vi "STD溶解氧_获取温度和测量值.vi"(5 "大气压补偿":dbl=1.0, 7 "盐度补偿":dbl, 8 "error in (no error)":errorcluster caption="错误输入（无错误）", 11 "MB session in":refnum<class "MB_Master.lvclass">) -> (0 "error out":errorcluster caption="错误输出", 2 "输出值":cluster{"温度测量值":sgl, "DO%":sgl, "DOmg/L":sgl}, 3 "MB session out":refnum<class "MB_Master.lvclass">)   [LabVIEW 2016, in "斯坦道多参数.lvlib"]
uses:
  <vilib>/Plasmionique/MB Master/MB_Master/MB_Master.lvclass
  <vilib>/Plasmionique/MB Master/MB Master.lvlib
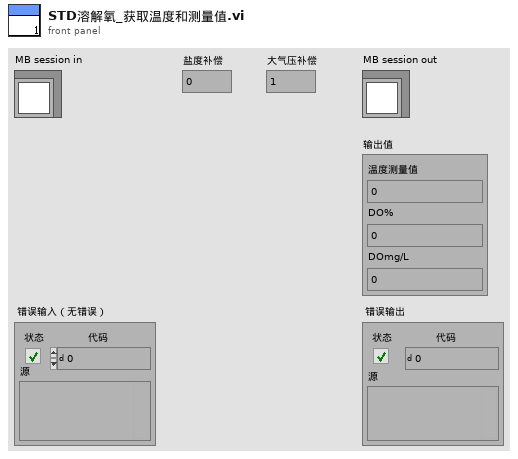
[diagram p1: front panel]
types:
  T1 = cluster{"pH":u32, "DO":u32, "Cond":u32, "Turb":u32, "叶绿素a":u32, "藻密度":u32, "ORP":u32, "COD":u32, "氯化物":u32, "氨氮":u32, "水中油":u32}
  T2 = cluster{"取值输出":dbl, "取值输出":dbl, "DataDo_mgL":dbl}
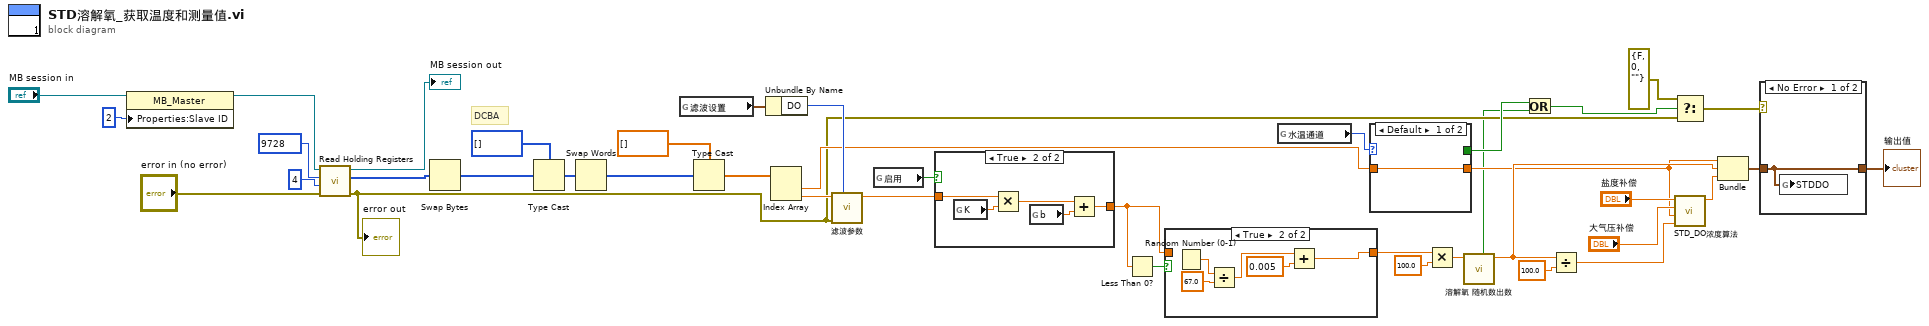
[diagram p0: block diagram]
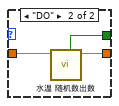
[diagram p4: hidden frame]
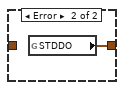
[diagram p5: hidden frame]
diagram:
  # "DCBA"
  n1 = property class="MB_Master"(reference="MB session in", "Properties:Slave ID"=u16 2 ("salve ID")) -> (reference out=w33:refnum<class "MB_Master.lvclass">)  [unwired: 1 in, 1 out]
  n2 = call <vilib>:"Read Holding Registers.vi"("error in (no error)"="error in (no error)", "quantity"=u16 4, "starting address"=u16 9728, "MB session in"=w33) -> ("error out"=w7:errorcluster, "Registers"=w32:u16[], "MB session out"=→"MB session out":refnum<class "MB_Master.lvclass">)  [unwired: 5 in]
  "error out" <- w7
  n3 = Swap Bytes(anything=w32) -> (byte swapped=w31:u16[])
  n4 = Type Cast(type=u32[] [] ("数组 2"), x=w31) -> (*(type *) &x=w37:u32[])
  n5 = Swap Words(1:w37) -> (0:w39:u32[])
  n6 = global read "断电保存变量.vi" "滤波设置"() -> (w23:T1)
  n7 = Type Cast(type=sgl[] [] ("数组 2"), x=w39) -> (*(type *) &x=w35:sgl[])
  n8 = Unbundle By Name(w23) -> ("DO"=w22:u32)
  n9 = Index Array(array=w35) -> (element #1=w11:sgl, element #2=w24:sgl)  [unwired: 2 in]
  n10 = call "滤波参数.vi"("滤波次数"=w22, "error in (no error)"=w7, "x"=w24) -> ("mode"=w5:dbl)  [unwired: 7 in, 1 out]
  n11 = global read "断电保存变量.vi" "启用"() -> (w6:bool)
  n12 = case shown="True" w6 {
    tunnel: w5 -> [w42 w47]
    tunnel: [w42 w43] -> w1
    frame False {
    }
    frame True {
      n13 = global read "断电保存变量.vi" "K"() -> (w46:dbl)
      n14 = Multiply(x=w47, y=w46) -> (x*y=w45:dbl)
      n15 = global read "断电保存变量.vi" "b"() -> (w44:dbl)
      n16 = Add(x=w45, y=w44) -> (x+y=w43:dbl)
    }
  }
  n17 = Less Than 0?(x=w1) -> (x < 0?=w3:bool)
  n18 = case shown="True" w3 {
    tunnel: [w48 w49] -> w2
    tunnel: w1 -> [w48 _]
    frame False {
    }
    frame True {
      n19 = Random Number (0-1)() -> (number: 0 to 1=w51:dbl)
      n20 = Divide(x=w51, y=67.0) -> (x/y=w52:dbl)
      n21 = Add(x=w52, y=0.005) -> (x+y=w49:dbl)
    }
  }
  n22 = global read "断电保存变量.vi" "水温通道"() -> (w12:enum16{"pH", "DO", "浊度", "电导率", "叶绿素a", "藻密度"})
  n23 = case shown="Default" w12 {
    tunnel: w11 -> [w54 w56]
    tunnel: [w54 w55] -> w10
    tunnel: [_ w57] -> w8
    frame Default {
    }
    frame "DO" {
      n24 = call "水温 随机数出数.vi"("原始值"=w56) -> ("取值输出"=w55:dbl, "x .and. y?"=w57:bool)  [unwired: 6 in, 1 out]
    }
  }
  n25 = Multiply(x=w2, y=100.0) -> (x*y=w17:dbl)
  n26 = call "溶解氧 随机数出数.vi"("原始值"=w17) -> ("取值输出"=w15:dbl, "x .and. y?"=w4:bool)  [unwired: 6 in, 1 out]
  n27 = Or(x=w8, y=w4) -> (x .or. y?=w9:bool)
  n28 = Divide(x=w15, y=100.0) -> (x/y=w14:dbl)
  n29 = Select(t=errorcluster {"status"=FALSE, "code"=0, "source"=""}, s=w9, f=w7) -> (s? t:f=w19:errorcluster)
  n30 = call "STD_DO浓度算法.vi"("溶解氧饱和度值"=w14, "水温"=w10, "大气压补偿"="大气压补偿", "盐度补偿"="盐度补偿") -> ("DataDo_mgL"=w30:dbl)  [unwired: 7 in]
  n31 = Bundle("取值输出"=w10, "取值输出"=w15, "DataDo_mgL"=w30) -> (w27:T2)  [unwired: 1 in]
  n32 = case shown="No Error" w19 {
    tunnel: w27 -> [w58 _]
    tunnel: [w58 w59] -> w21
    frame No Error {
      n33 = global write "禹山过程全局变量.vi" "STDDO"(w58) -> ()
    }
    frame Error {
      n34 = global read "禹山过程全局变量.vi" "STDDO"() -> (w59:cluster{"温度测量值":sgl, "DO%":sgl, "DOmg/L":sgl})
    }
  }
  "输出值" <- w21
